vi "MoveGantry.vi"(8 "error in (no error)":errorcluster, 10 "targetPosn [xyz]":T1, 11 "Axis List In [xyz]":refnum<class "Axis.lvclass">[](array[class])) -> (0 "error out":errorcluster, 3 "Axis List In [xyz] 2":refnum<class "Axis.lvclass">[](array[class]))   [LabVIEW 2020]
uses:
  Axis.lvclass
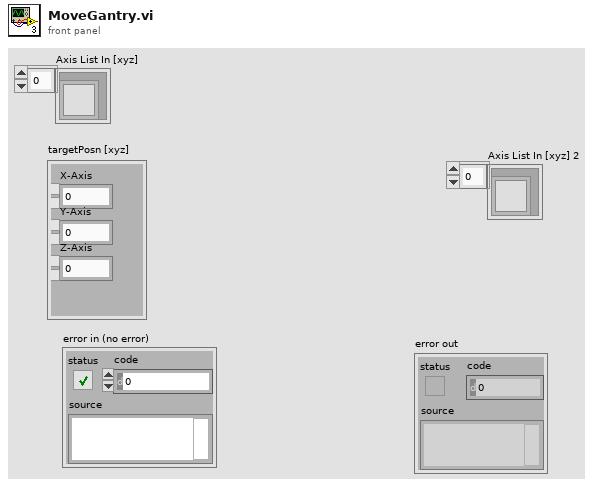
[diagram p1: front panel]
types:
  T1 = cluster{"X-Axis":i32, "Y-Axis":i32, "Z-Axis":i32}
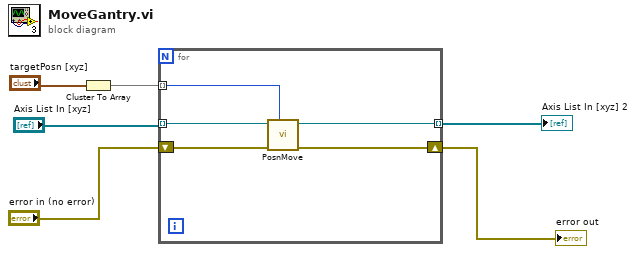
[diagram p0: block diagram]
diagram:
  n1 = Cluster To Array(cluster="targetPosn [xyz]") -> (array=w5:i32[])
  n2 = for {
    tunnel: "Axis List In [xyz]" -> [w11] mode=indexing
    tunnel: w5 -> [w10] mode=indexing
    shift-right: [w8] -> w2
    shift-left: "error in (no error)" -> [w9]
    tunnel: [w7] -> w1 mode=indexing
    n3 = call "PosnMove.vi"("targetPosn"=w10, "error in (no error)"=w9, "Axis in"=w11) -> ("error out"=w8:errorcluster, "Axis out"=w7:refnum<class "Axis.lvclass">)  [unwired: 7 in]
  }
  "error out" <- w2
  "Axis List In [xyz] 2" <- w1
